vi "Periodic Tasks.vi"(8 "error in":errorcluster) -> ()   [LabVIEW 2018]
doc: "This VI runs in parallel to other tasks. It can contain as many user-defined periodic loops as you need. These can carry out PID or other sorts of timed response."
uses:
  <vilib>/Rock Robotics/WPI/ThirdParty/sensors/navX/_TypeDefs/Flags/Z900_navX_Flags_OpStatusTypeDef.ctl
  <vilib>/Rock Robotics/WPI/ThirdParty/sensors/navX/_TypeDefs/Flags/Z900_navX_Flags_CalibrationStatusTypeDef.ctl
  SwerveRotationCalibrate.ctl
  <vilib>/Rock Robotics/WPI/ThirdParty/Phoenix-LabVIEW/Motor Controller/Controls/CTRE_Phoenix_MotorControl_NeutralMode.ctl
  <vilib>/Rock Robotics/WPI/ThirdParty/Phoenix-LabVIEW/Motor Controller/Controls/CTRE_Phoenix_MotorControl_ControlMode.ctl
  <vilib>/Rock Robotics/WPI/ThirdParty/Phoenix-LabVIEW/Motor Controller/Controls/CTRE_Phoenix_MotorControl_FeedbackDevice.ctl
  HatchModes.ctl
  ElevBasePos.ctl
  ElevModes.ctl
  SequenceActions.ctl
  d8969dce-e83f-414b-ab1b-b6caec8a5545.vi
  83e91fab-fc29-4c7d-8b1e-156214dcbbb8.vi
  a102eae3-c5ed-494b-96cc-72fbbd712b4d.vi
  <vilib>/Rock Robotics/WPI/Utilities/WPI_GetSetVariantRefNum.vi
  <vilib>/Rock Robotics/Network Tables/NT Read Boolean.vi
  Robot Global Data.vi
  <vilib>/Rock Robotics/Network Tables/NT Write Number.vi
  <vilib>/Rock Robotics/Network Tables/NT Write String.vi
  <vilib>/Rock Robotics/Network Tables/NT Write Boolean.vi
panel:
  in  "Calibration Status":T1=3 items=["IMU_CAL_STATE_MASK"=3, "IMU_CAL_STATE_INPROGRESS"=0, "IMU_CAL_STATE_ACCUMULATE"=1, "IMU_CAL_STATE_COMPLETE"=2]
  in  "OP Status":T2 items=["INITIALIZING", "SELFTEST_IN_PROGRESS", "ERROR", "IMU_AUTOCAL_IN_PROGRESS", "NORMAL"]
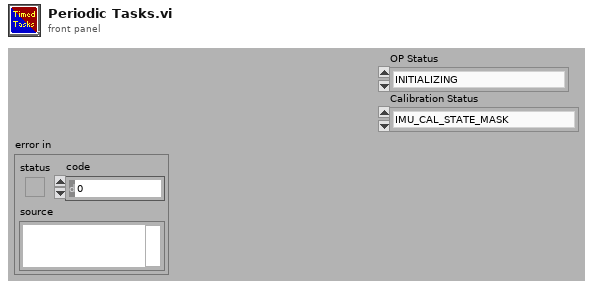
[diagram p1: front panel]
types:
  T1 = typedef "Z900_navX_Flags_CalibrationStatusTypeDef.ctl" = u8
  T2 = typedef "Z900_navX_Flags_OpStatusTypeDef.ctl" = u8
  T3 = typedef "HatchModes.ctl" = enum16{"Travel", "PickPlaceShip", "PlaceRocket"}
  T4 = typedef "SwerveRotationCalibrate.ctl" = enum16{"Calibrate", "Home", "ManualHome", "ResetQuad", "Drive"}
  T5 = typedef "CTRE_Phoenix_MotorControl_NeutralMode.ctl" = enum8{"EEPROMSetting", "Override to Coast", "Override to Brake"}
  T6 = typedef "CTRE_Phoenix_MotorControl_ControlMode.ctl" = u16
  T7 = typedef "CTRE_Phoenix_MotorControl_FeedbackDevice.ctl" = i8
  T8 = cluster{"T0":u32, "Mode":T4, "Rotation Neutral Mode":T5, "Rotation Control Mode":T6, "Feedback Device":T7}
  T9 = cluster{"Update Rate Hz":u8, "Accelerometer Full-Scale Range":u8, "Gyro Full-Scale Range":u16, "OP Status":T2, "Calibration Status":T1, "Sensor Status":cluster{"MOVING":bool, "YAW_STABLE":bool, "MAG_DISTURBANCE":bool, "ALTITUDE_VALID":bool, "SEALEVEL_PRESS_SET":bool, "FUSED_HEADING_VALID":bool}, "Self Test Status":cluster{"Gyro Passed":bool, "Accel Passed":bool, "Mag Passed":bool, "Baro Passed":bool, "Complete":bool}}
  T10 = typedef "ElevModes.ctl" = enum16{"Manual", "Auto"}
  T11 = typedef "ElevBasePos.ctl" = enum16{"NoChange", "ShipHatch", "RocketHatch", "Carry", "Cargo"}
  T12 = typedef "WPI_JoystickDevRef.ctl" = cluster{"Device":T13}
  T13 = typedef "WPI_JoystickDeviceEnum.ctl" = enum16{"USB 0", "USB 1", "USB 2", "USB 3", "USB 4", "USB 5"}
  T14 = typedef "SequenceActions.ctl" = enum16{"HatchLatch", "MoveElev", "Ready"}
  T15 = typedef "WPI_DriverStationRobotMode2.ctl" = enum16{"Autonomous Disabled", "Autonomous Enabled", "Teleop Disabled", "Teleop Enabled", "Disconnected", "Finish", "Test Disabled", "Test Enabled", "Emergency Stopped"}
  T16 = cluster{"Buttons[0]":bool, "Buttons[1]":bool, "Buttons[2]":bool, "Buttons[3]":bool, "Buttons[4]":bool, "Buttons[5]":bool, "Buttons[6]":bool, "Buttons[7]":bool, "Buttons[8]":bool, "Buttons[9]":bool, "Buttons[10]":bool, "Buttons[11]":bool, "Buttons[12]":bool}
  T17 = cluster{"Motor1":cluster{"P":dbl, "I":dbl, "D":dbl}, "Motor3":cluster{"P":dbl, "I":dbl, "D":dbl}, "Motor2":cluster{"P":dbl, "I":dbl, "D":dbl}, "Motor4":cluster{"P":dbl, "I":dbl, "D":dbl}}
  T18 = typedef "WPI_CompressorDevRef.ctl" = cluster{"DevStatus":errorcluster, "Pneumatics Control Module":u8}
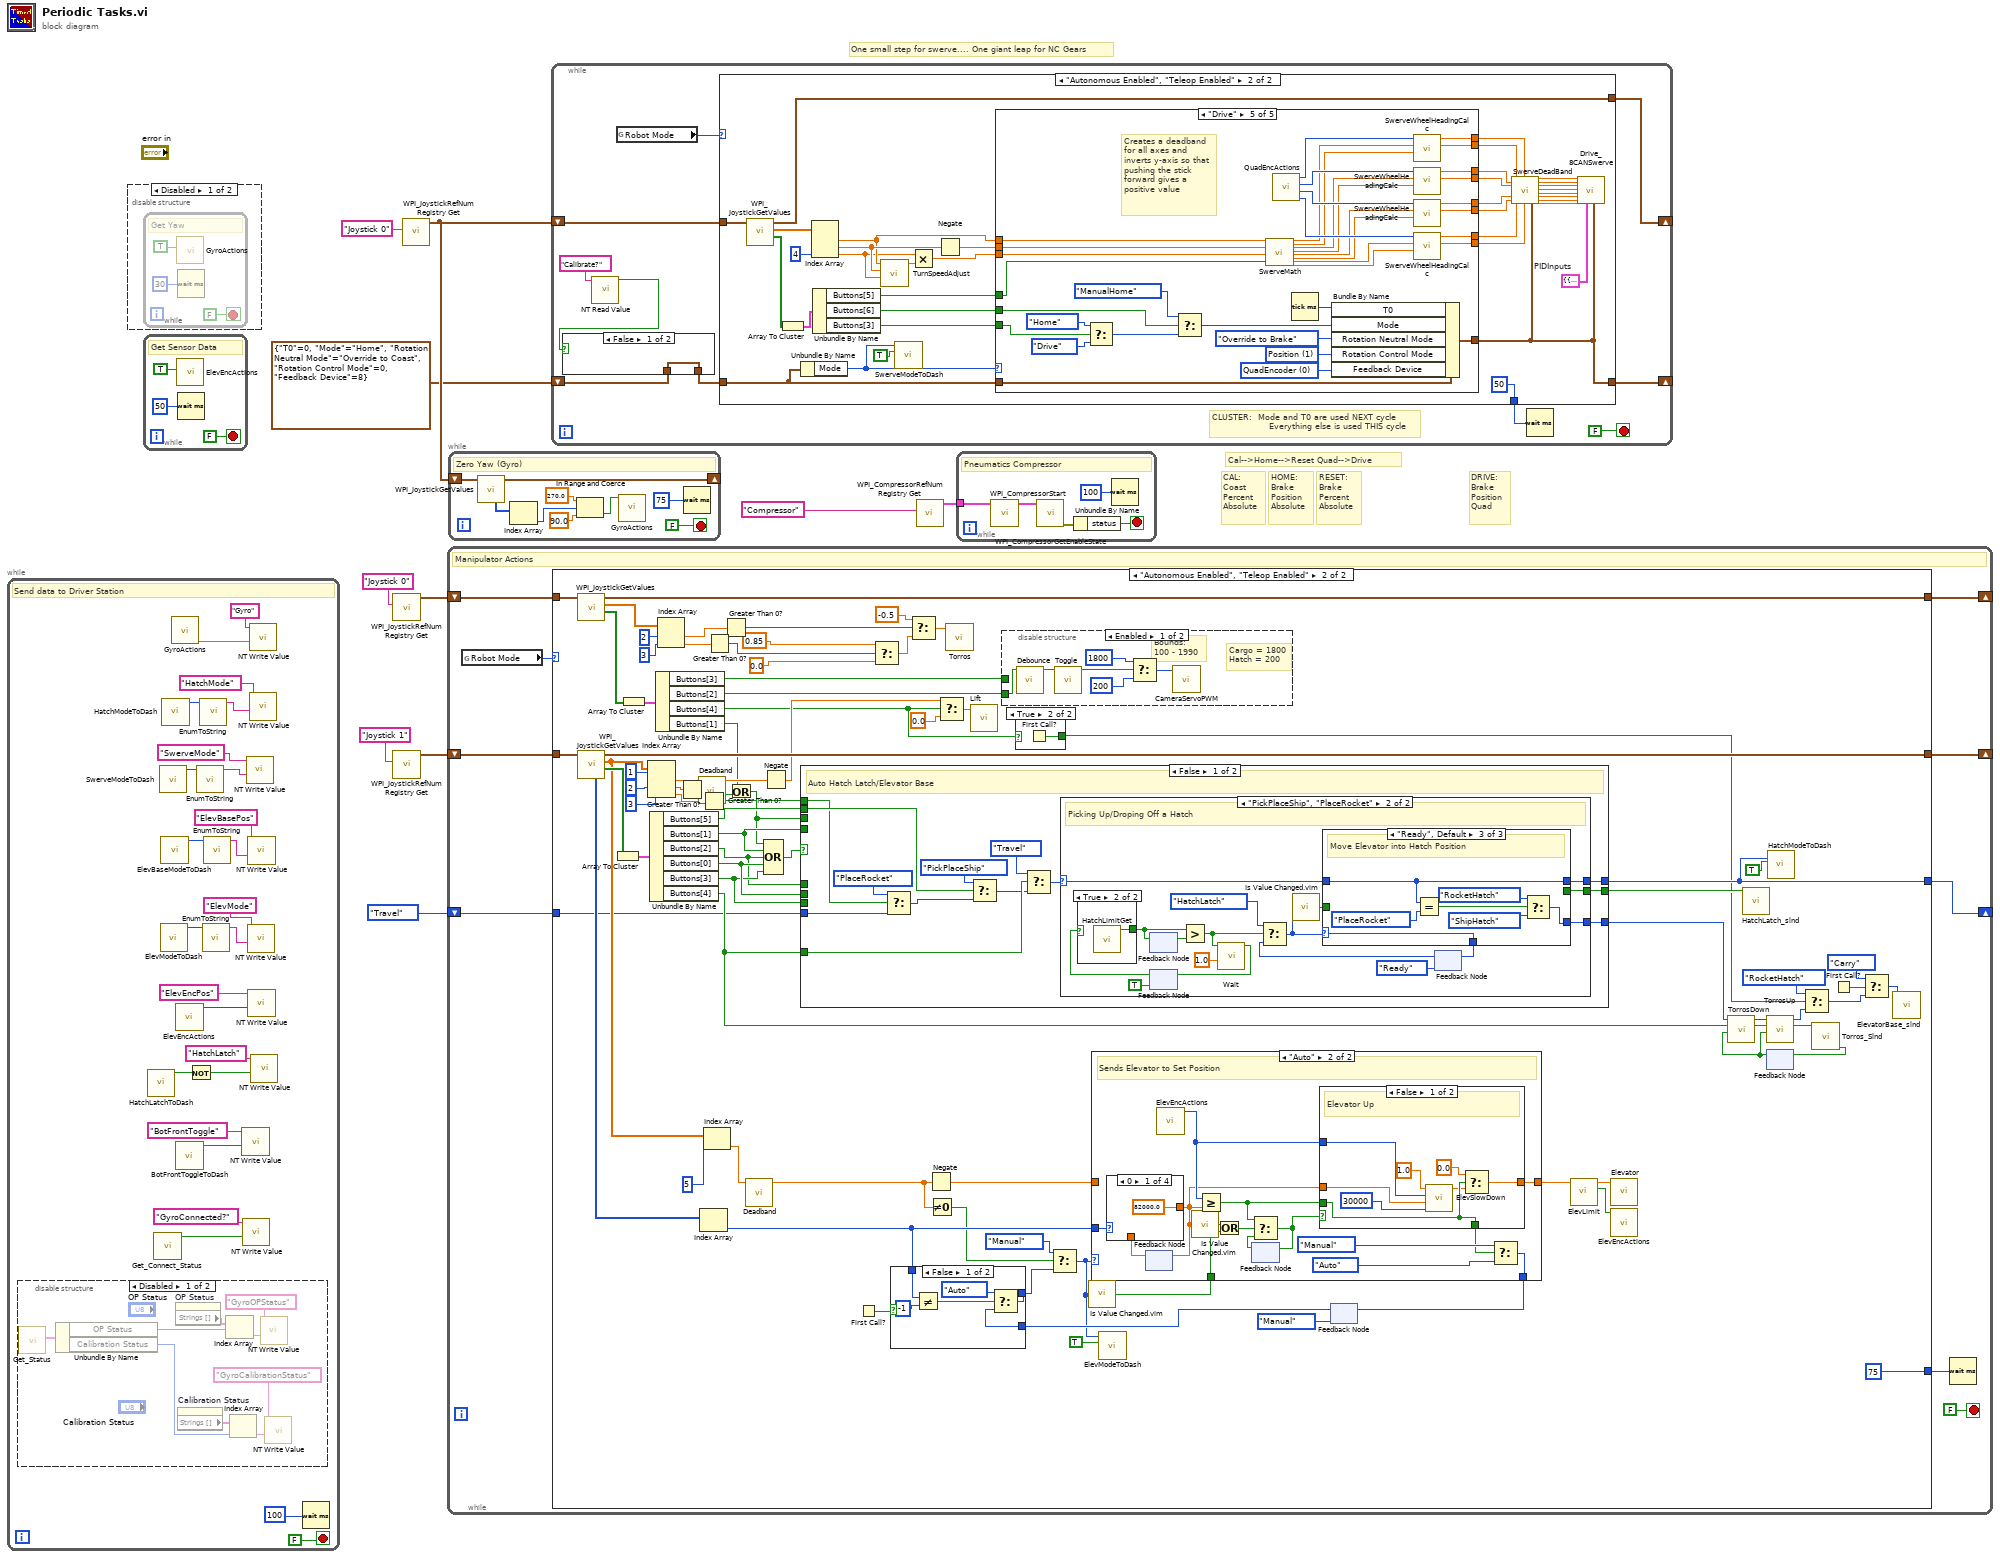
[diagram p0: block diagram]
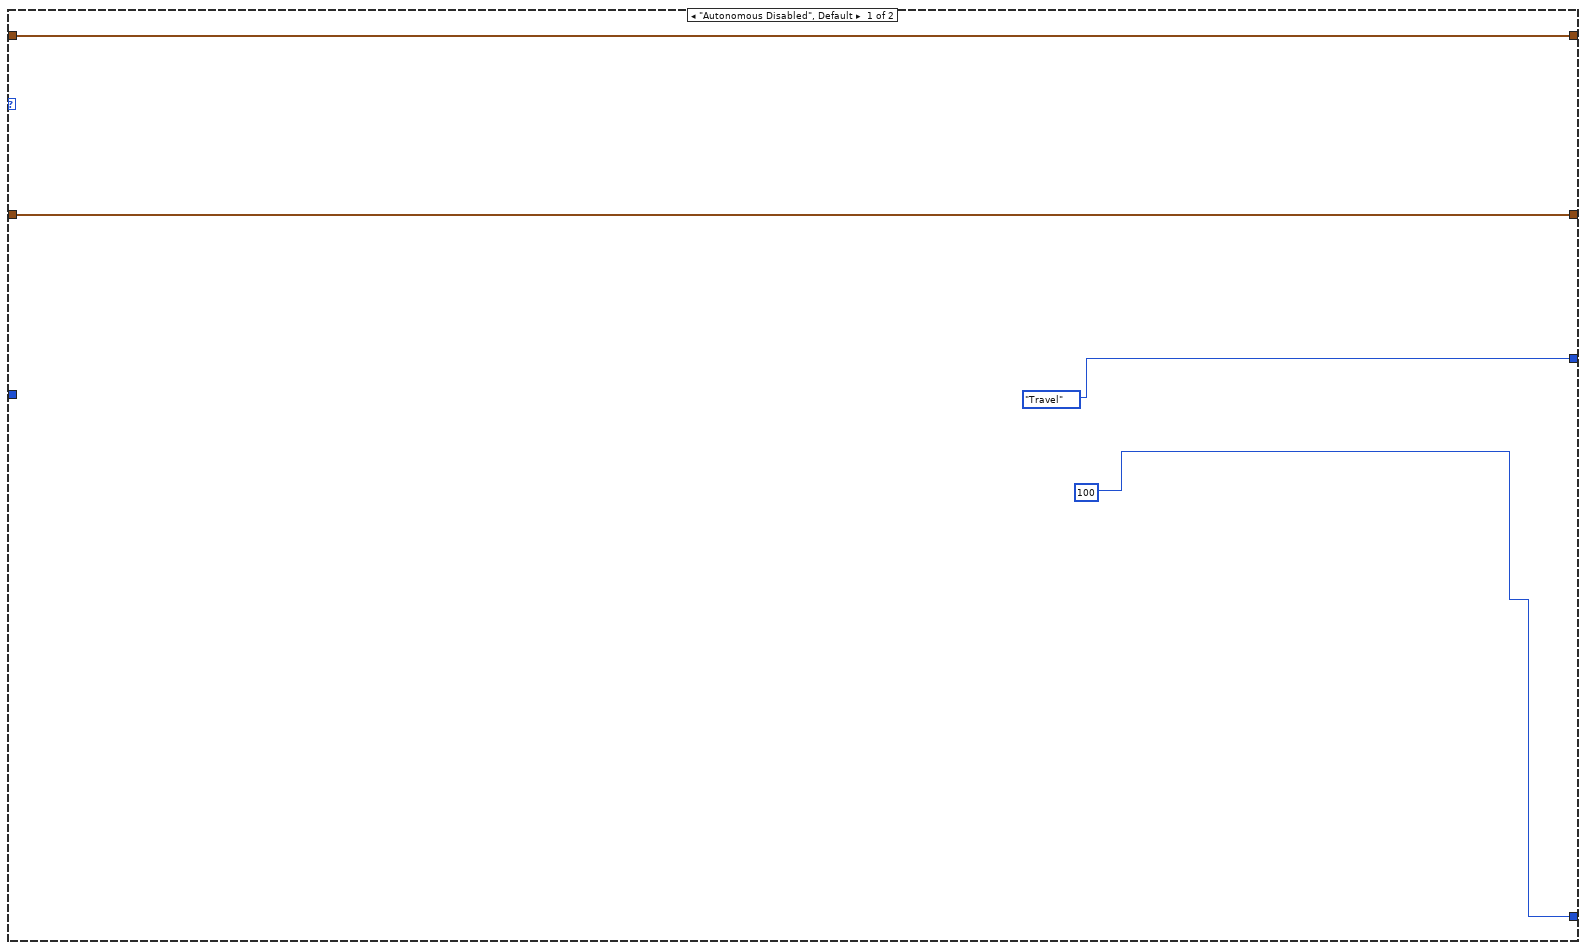
[diagram p3: hidden frame]
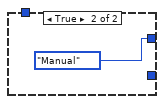
[diagram p4: hidden frame]
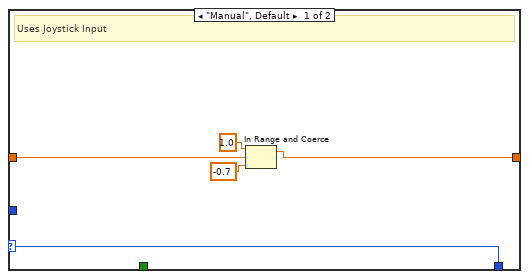
[diagram p5: hidden frame]
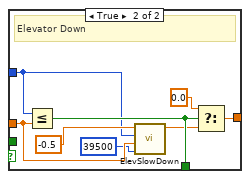
[diagram p6: hidden frame]
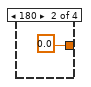
[diagram p7: hidden frame]
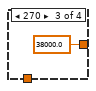
[diagram p8: hidden frame]
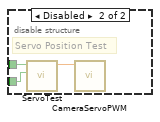
[diagram p11: hidden frame]
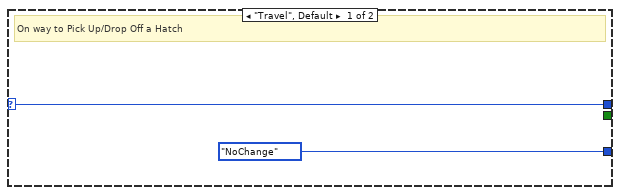
[diagram p12: hidden frame]
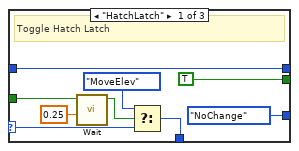
[diagram p14: hidden frame]
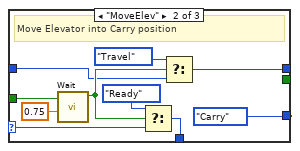
[diagram p15: hidden frame]
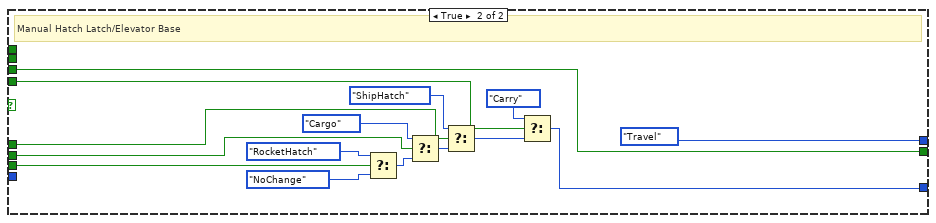
[diagram p16: hidden frame]
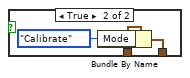
[diagram p17: hidden frame]
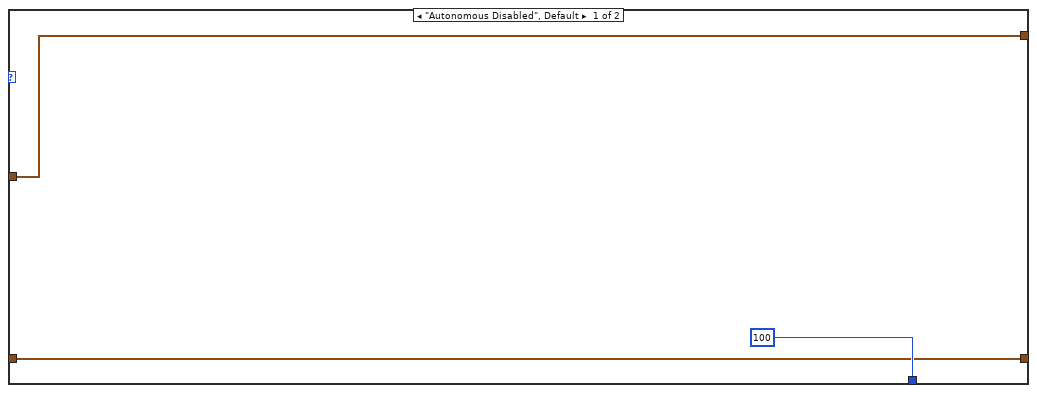
[diagram p18: hidden frame]
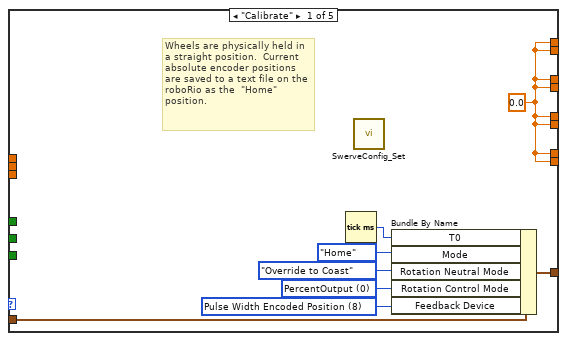
[diagram p19: hidden frame]
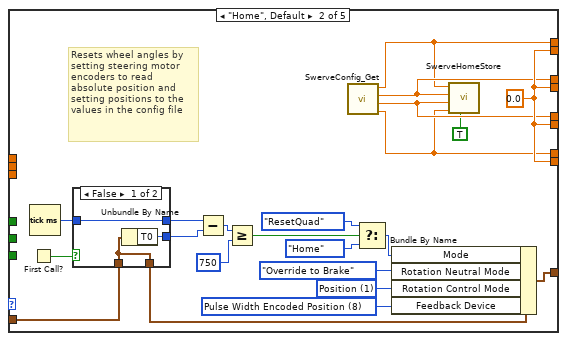
[diagram p20: hidden frame]
diagram:
  # "One small step for swerve.... One giant leap for NC Gears"
  # "DRIVE:\nBrake\nPosition\nQuad"
  # "RESET:\nBrake\nPercent\nAbsolute"
  # "HOME:\nBrake\nPosition\nAbsolute"
  # "Cal-->Home-->Reset Quad-->Drive"
  # "CAL:\nCoast\nPercent\nAbsolute"
  n1 = while {
    stop <- FALSE stop-if-true
    # "Send data to Driver Station"
    n2 = disable-structure shown="Disabled" {
      frame Disabled {
        n3 = call <vilib>:"Get_Status.vi"() -> ("Status"=w42:T9)  [unwired: 11 in]
        n4 = Unbundle By Name(w42) -> ("OP Status"=w40:T2, "Calibration Status"=w38:T1)
        n5 = property on="OP Status" class="Ring (strict)"() -> ("Strings []"=w41:string[])  [unwired: 2 in, 2 out]
        n6 = property on="Calibration Status" class="Ring (strict)"() -> ("Strings []"=w37:string[])  [unwired: 2 in, 2 out]
        n7 = Index Array(array=w41, index=w40) -> (element=w39:string)
        n8 = Index Array(array=w37, index=w38) -> (element=w36:string)
        n9 = call-poly <vilib>:"NT Write Value.vi"("String"=w39, "Name"="GyroOPStatus") -> ()  [unwired: 9 in, 1 out]
        n10 = call-poly <vilib>:"NT Write Value.vi"("String"=w36, "Name"="GyroCalibrationStatus") -> ()  [unwired: 9 in, 1 out]
      }
      frame Enabled {
      }
    }
    n11 = call "HatchLatchToDash.vi"() -> ("HatchLatchOut"=w11:bool)  [unwired: 11 in]
    n12 = call <vilib>:"Get_Connect_Status.vi"() -> ("Connected"=w19:bool)  [unwired: 11 in]
    n13 = call "SwerveModeToDash.vi"() -> ("SwerveModeOut"=w27:T4)  [unwired: 11 in]
    n14 = call "ElevModeToDash.vi"() -> ("ElevModeOut"=w17:T10)  [unwired: 11 in]
    n15 = call "ElevBaseModeToDash.vi"() -> ("ElevBasePosOut"=w22:T11)  [unwired: 11 in]
    n16 = call "HatchModeToDash.vi"() -> ("HatchModeOut"=w30:T3)  [unwired: 11 in]
    n17 = call "GyroActions.vi"() -> ("Yaw"=w18:dbl)  [unwired: 10 in, 1 out]
    n18 = call "ElevEncActions.vi"() -> ("ElevEncPos"=w24:i32)  [unwired: 11 in]
    n19 = call "BotFrontToggleToDash.vi"() -> ("FrontToggleOut"=w14:bool)  [unwired: 11 in]
    n20 = Not(x=w11) -> (.not. x?=w12:bool)
    n21 = call "EnumToString.vi"("Enum"=w27) -> ("String"=w26:string)  [unwired: 10 in]
    n22 = call "EnumToString.vi"("Enum"=w30) -> ("String"=w29:string)  [unwired: 10 in]
    n23 = call "EnumToString.vi"("Enum"=w17) -> ("String"=w16:string)  [unwired: 10 in]
    n24 = call "EnumToString.vi"("Enum"=w22) -> ("String"=w31:string)  [unwired: 10 in]
    n25 = call-poly <vilib>:"NT Write Value.vi"("Boolean"=w14, "Name"="BotFrontToggle") -> ()  [unwired: 9 in, 1 out]
    n26 = call-poly <vilib>:"NT Write Value.vi"("Boolean"=w19, "Name"="GyroConnected?") -> ()  [unwired: 9 in, 1 out]
    n27 = call-poly <vilib>:"NT Write Value.vi"("String"=w26, "Name"="SwerveMode") -> ()  [unwired: 9 in, 1 out]
    n28 = call-poly <vilib>:"NT Write Value.vi"("String"=w16, "Name"="ElevMode") -> ()  [unwired: 9 in, 1 out]
    n29 = call-poly <vilib>:"NT Write Value.vi"("String"=w31, "Name"="ElevBasePos") -> ()  [unwired: 9 in, 1 out]
    n30 = call-poly <vilib>:"NT Write Value.vi"("Numeric"=w24, "Name"="ElevEncPos") -> ()  [unwired: 9 in, 1 out]
    n31 = call-poly <vilib>:"NT Write Value.vi"("Numeric"=w18, "Name"="Gyro") -> ()  [unwired: 9 in, 1 out]
    n32 = call-poly <vilib>:"NT Write Value.vi"("String"=w29, "Name"="HatchMode") -> ()  [unwired: 9 in, 1 out]
    n33 = call-poly <vilib>:"NT Write Value.vi"("Boolean"=w12, "Name"="HatchLatch") -> ()  [unwired: 9 in, 1 out]
    n34 = Wait (ms)(milliseconds to wait=u32 100 ("millisecond timer value")) -> ()  [unwired: 1 out]
  }
  n35 = disable-structure shown="Disabled" {
    frame Disabled {
      n36 = while {
        stop <- FALSE stop-if-true
        # "Get Yaw"
        n37 = call "GyroActions.vi"("Update?"=TRUE ("Zero")) -> ()  [unwired: 9 in, 2 out]
        n38 = Wait (ms)(milliseconds to wait=u32 30) -> ()  [unwired: 1 out]
      }
    }
    frame Enabled {
    }
  }
  n39 = while {
    stop <- FALSE stop-if-true
    # "Get Sensor Data"
    n40 = call "ElevEncActions.vi"("Update?"=TRUE ("Zero")) -> ()  [unwired: 10 in, 1 out]
    n41 = Wait (ms)(milliseconds to wait=u32 50) -> ()  [unwired: 1 out]
  }
  n42 = call <vilib>:"WPI_JoystickRefNum Registry Get.vi"("refnum name"="Joystick 0") -> ("JoystickDevRef"=w2:T12)  [unwired: 1 in, 9 out]
  n43 = call <vilib>:"WPI_JoystickRefNum Registry Get.vi"("refnum name"="Joystick 1") -> ("JoystickDevRef"=w6:T12)  [unwired: 1 in, 9 out]
  n44 = call <vilib>:"WPI_JoystickRefNum Registry Get.vi"("refnum name"="Joystick 0") -> ("JoystickDevRef"=w9:T12)  [unwired: 1 in, 9 out]
  n45 = while {
    shift-right: [w53] -> _
    shift-left: HatchModes."Travel" -> [w54]
    shift-right: [w52] -> _
    shift-left: w6 -> [w58]
    shift-right: [w51] -> _
    shift-left: w2 -> [w55]
    stop <- FALSE stop-if-true
    # "Manipulator Actions"
    n46 = global read "Robot Global Data.vi" "Robot Mode"() -> (w59:T15)
    n47 = case shown="\"Autonomous Enabled\", \"Teleop Enabled\"" w59 {
      tunnel: w58 -> [w61 w144]
      tunnel: [u32 100 ("milliseconds to wait") u32 75 ("milliseconds to wait")] -> w56
      tunnel: w55 -> [w60 w138]
      tunnel: w54 -> [_ w93]
      tunnel: [HatchModes."Travel" w106] -> w53
      tunnel: [w61 w101] -> w52
      tunnel: [w60 w64] -> w51
      frame "Autonomous Disabled", Default {
      }
      frame "Autonomous Enabled", "Teleop Enabled" {
        n48 = call <vilib>:"WPI_JoystickGetValues.vi"("JoystickDevRef"=w138) -> ("Buttons"=w139:bool[], "Axes"=w128:dbl[], "JoystickDevRef"=w64:T12)  [unwired: 6 in, 2 out]
        n49 = call <vilib>:"WPI_JoystickGetValues.vi"("JoystickDevRef"=w144) -> ("Buttons"=w143:bool[], "Axes"=w102:dbl[], "JoystickDevRef"=w101:T12, "POVs"=w141:i16[])  [unwired: 6 in, 1 out]
        n50 = Array To Cluster(array=w143) -> (cluster=w145:T16)
        n51 = Array To Cluster(array=w139) -> (cluster=w140:T16)
        n52 = Index Array(array=w102, index #1=1 ("index"), index #2=2 ("index"), index #3=3 ("index")) -> (element #1=w100:dbl, element #2=w89:dbl, element #3=w70:dbl)
        n53 = Unbundle By Name(w145) -> ("Buttons[5]"=w114:bool, "Buttons[1]"=w136:bool, "Buttons[2]"=w104:bool, "Buttons[0]"=w135:bool, "Buttons[3]"=w134:bool, "Buttons[4]"=w94:bool)
        n54 = Unbundle By Name(w140) -> ("Buttons[3]"=w91:bool, "Buttons[2]"=w92:bool, "Buttons[4]"=w84:bool, "Buttons[1]"=w65:bool)
        n55 = Index Array(array=w128, index #1=2 ("index"), index #2=3 ("index")) -> (element #1=w124:dbl, element #2=w125:dbl)
        n56 = Greater Than 0?(x=w89) -> (x > 0?=w88:bool)
        n57 = call "Deadband.vi"("Input"=w100) -> ("Output"=w71:dbl)  [unwired: 6 in]
        n58 = Index Array(array=w141) -> (element=w130:i16)  [unwired: 1 in]
        n59 = Greater Than 0?(x=w70) -> (x > 0?=w69:bool)
        n60 = Index Array(array=w102, index=5) -> (element=w115:dbl)
        n61 = Greater Than 0?(x=w125) -> (x > 0?=w122:bool)
        n62 = Greater Than 0?(x=w124) -> (x > 0?=w123:bool)
        n63 = Or(x=w65, y=w88) -> (x .or. y?=w87:bool)
        n64 = call "Deadband.vi"("Input"=w115) -> ("Output"=w132:dbl)  [unwired: 6 in]
        n65 = Negate(x=w71) -> (-x=w98:dbl)
        n66 = Compound Arithmetic op=OR(w87, w136, w104, w135, w134) -> (w137:bool)
        n67 = case shown="False" w137 {
          tunnel: w93 -> [w205 _]
          tunnel: [w215 HatchModes."Travel"] -> w106
          tunnel: [w214 w275] -> w133
          tunnel: w87 -> [_ w275]
          tunnel: w136 -> [_ w274]
          tunnel: w104 -> [_ w273]
          tunnel: w135 -> [_ w272]
          tunnel: w134 -> [_ w271]
          tunnel: w114 -> [w212 _]
          tunnel: [w211 w262] -> w111
          tunnel: w94 -> [w210 _]
          tunnel: w69 -> [w203 _]
          frame False {
            # "Auto Hatch Latch/Elevator Base"
            n68 = Select(t=HatchModes."PlaceRocket", s=w203, f=w205) -> (s? t:f=w204:T3)
            n69 = Select(t=HatchModes."PickPlaceShip", s=w212, f=w204) -> (s? t:f=w208:T3)
            n70 = Select(t=HatchModes."Travel", s=w210, f=w208) -> (s? t:f=w207:T3)
            n71 = case shown="\"PickPlaceShip\", \"PlaceRocket\"" w207 {
              selector: w207 -> [w217 w234]
              tunnel: [w217 w233] -> w215
              tunnel: [_ w232] -> w214
              tunnel: [ElevBasePos."NoChange" w225] -> w211
              frame "Travel", Default {
                # "On way to Pick Up/Drop Off a Hatch"
              }
              frame "PickPlaceShip", "PlaceRocket" {
                # "Picking Up/Droping Off a Hatch"
                n72 = feedback #1() -> (w220:bool)  [unwired: 1 in]
                n73 = feedback #2(TRUE ("Completed")) -> (w222:bool)
                n74 = case shown="True" w222 {
                  tunnel: [_ w235] -> w218
                  frame False {
                  }
                  frame True {
                    n75 = call "HatchLimitGet.vi"() -> ("Pressed?"=w235:bool)  [unwired: 11 in]
                  }
                }
                n76 = feedback-in #1(w218) -> ()
                n77 = Greater?(x=w218, y=w220) -> (0:w219:bool)
                n78 = call "Wait.vi"("Target Time (s)"=1.0, "Start Timer?"=w219) -> ("Completed"=w223:bool)  [unwired: 8 in, 1 out]
                n79 = feedback-in #2(w223) -> ()
                n80 = feedback #3(SequenceActions."Ready" ("SequenceAction")) -> (w229:T14)
                n81 = Select(t=SequenceActions."HatchLatch" ("SequenceAction"), s=w219, f=w229) -> (s? t:f=w231:T14)
                n82 = call "Is Value Changed.vim"("value"=w231) -> ("changed or first call?"=w226:bool)
                n83 = case shown="\"Ready\", Default" w231 {
                  selector: w231 -> [w243 w254 w261]
                  tunnel: [w242 w253 w261] -> w230
                  tunnel: w234 -> [w241 w250 w255]
                  tunnel: [w241 w249 w255] -> w233
                  tunnel: [TRUE _ _] -> w232
                  tunnel: w226 -> [w238 w247 _]
                  tunnel: [ElevBasePos."NoChange" ElevBasePos."Carry" w258] -> w225
                  frame "HatchLatch" {
                    # "Toggle Hatch Latch"
                    n84 = call "Wait.vi"("Target Time (s)"=0.25, "Start Timer?"=w238) -> ("Completed"=w244:bool)  [unwired: 8 in, 1 out]
                    n85 = Select(t=SequenceActions."MoveElev" ("SequenceAction"), s=w244, f=w243) -> (s? t:f=w242:T14)
                  }
                  frame "MoveElev" {
                    # "Move Elevator into Carry position"
                    n86 = call "Wait.vi"("Target Time (s)"=0.75, "Start Timer?"=w247) -> ("Completed"=w252:bool)  [unwired: 8 in, 1 out]
                    n87 = Select(t=SequenceActions."Ready" ("SequenceAction"), s=w252, f=w254) -> (s? t:f=w253:T14)
                    n88 = Select(t=HatchModes."Travel", s=w252, f=w250) -> (s? t:f=w249:T3)
                  }
                  frame "Ready", Default {
                    # "Move Elevator into Hatch Position"
                    n89 = Equal?(x=w255, y=HatchModes."PlaceRocket") -> (x = y?=w257:bool)
                    n90 = Select(t=ElevBasePos."RocketHatch", s=w257, f=ElevBasePos."ShipHatch") -> (s? t:f=w258:T11)
                  }
                }
                n91 = feedback-in #3(w230) -> ()
              }
            }
          }
          frame True {
            # "Manual Hatch Latch/Elevator Base"
            n92 = Select(t=ElevBasePos."RocketHatch", s=w271, f=ElevBasePos."NoChange") -> (s? t:f=w270:T11)
            n93 = Select(t=ElevBasePos."Cargo", s=w272, f=w270) -> (s? t:f=w269:T11)
            n94 = Select(t=ElevBasePos."ShipHatch", s=w273, f=w269) -> (s? t:f=w268:T11)
            n95 = Select(t=ElevBasePos."Carry", s=w274, f=w268) -> (s? t:f=w262:T11)
          }
        }
        n96 = First Call?() -> (First Call?: T/F=w66:bool)
        n97 = Select(t=0.85, s=w122, f=0.0) -> (s? t:f=w121:dbl)
        n98 = Select(t=-0.5, s=w123, f=w121) -> (s? t:f=w120:dbl)
        n99 = Negate(x=w132) -> (-x=w75:dbl)
        n100 = Not Equal To 0?(x=w132) -> (x != 0?=w76:bool)
        n101 = Select(t=w98, s=w84, f=0.0 ("t")) -> (s? t:f=w86:dbl)
        n102 = call "Torros.vi"("Power"=w120) -> ()  [unwired: 11 in]
        n103 = call "Lift.vi"("Power"=w86) -> ()  [unwired: 11 in]
        n104 = disable-structure shown="Enabled" {
          disable-tunnel: w92 -> [w195 w202]
          disable-tunnel: w91 -> [_ w201]
          frame Enabled {
            # "Cargo = 1800\nHatch = 200"
            # "Bounds: 100 - 1990"
            n105 = call "Debounce.vi"("booleanIn"=w195) -> ("booleanOut"=w196:bool)  [unwired: 10 in]
            n106 = call "Toggle.vi"("booleanIn"=w196) -> ("booleanOut"=w197:bool)  [unwired: 10 in]
            n107 = Select(t=1800, s=w197, f=200) -> (s? t:f=w194:i32)
            n108 = call "CameraServoPWM.vi"("Position"=w194) -> ()  [unwired: 11 in]
          }
          frame Disabled {
            # "Servo Position Test"
            n109 = call "ServoTest.vi"("Down"=w202, "Up"=w201) -> ("Angle"=w200:dbl)  [unwired: 9 in]
            n110 = call "CameraServoPWM.vi"("Position"=w200) -> ()  [unwired: 11 in]
          }
        }
        n111 = case shown="True" w84 {
          tunnel: [_ w193] -> w83
          frame False {
          }
          frame True {
            n112 = First Call?() -> (First Call?: T/F=w193:bool)
          }
        }
        n113 = feedback #4(ElevModes."Manual") -> (w77:T10)
        n114 = case shown="False" w66 {
          tunnel: w130 -> [w151 _]
          tunnel: [w150 ElevModes."Manual"] -> w79
          tunnel: w77 -> [w148 _]
          frame False {
            n115 = Not Equal?(x=w151, y=i16 -1) -> (x != y?=w146:bool)
            n116 = Select(t=ElevModes."Auto", s=w146, f=w148) -> (s? t:f=w150:T10)
          }
          frame True {
          }
        }
        n117 = Select(t=ElevModes."Manual", s=w76, f=w79) -> (s? t:f=w68:T10)
        n118 = call "Is Value Changed.vim"("value"=w68) -> ("changed or first call?"=w74:bool)
        n119 = case shown="\"Auto\"" w68 {
          selector: w68 -> [w157 _]
          tunnel: w130 -> [_ w172]
          tunnel: [w155 w171] -> w131
          tunnel: w75 -> [w156 _]
          tunnel: w74 -> [_ w163]
          tunnel: [w157 w158] -> w73
          frame "Manual", Default {
            # "Uses Joystick Input"
            n120 = In Range and Coerce(upper limit=1.0, x=w156, lower limit=-0.7) -> (coerced(x)=w155:dbl)  [unwired: 1 out]
          }
          frame "Auto" {
            # "Sends Elevator to Set Position"
            n121 = feedback #5() -> (w166:dbl)  [unwired: 1 in]
            n122 = case shown="0" w172 {
              tunnel: [82000.0 ("Target") 0.0 ("Target") 38000.0 ("Target") w192] -> w165
              tunnel: w166 -> [_ _ _ w192]
              frame 0 {
              }
              frame 180 {
              }
              frame 270 {
              }
              frame -1, Default {
              }
            }
            n123 = feedback-in #5(w165) -> ()
            n124 = call "ElevEncActions.vi"() -> ("ElevEncPos"=w167:i32)  [unwired: 11 in]
            n125 = call "Is Value Changed.vim"("value"=w165) -> ("changed or first call?"=w164:bool)
            n126 = Greater Or Equal?(x=w167, y=w165) -> (x >= y?=w168:bool)
            n127 = Or(x=w164, y=w163) -> (x .or. y?=w162:bool)
            n128 = feedback #6() -> (w170:bool)  [unwired: 1 in]
            n129 = Select(t=w168, s=w162, f=w170) -> (s? t:f=w169:bool)
            n130 = feedback-in #6(w169) -> ()
            n131 = case shown="False" w169 {
              tunnel: [w179 w187] -> w171
              tunnel: w165 -> [w175 w183]
              tunnel: w167 -> [w176 w184]
              tunnel: w168 -> [w178 _]
              tunnel: [w178 w186] -> w159
              frame False {
                # "Elevator Up"
                n132 = call "ElevSlowDown.vi"("SlowRange"=30000 ("y"), "Target"=w175, "Current"=w176, "ElevIn"=1.0) -> ("ElevOut"=w174:dbl)  [unwired: 7 in]
                n133 = Select(t=0.0, s=w178, f=w174) -> (s? t:f=w179:dbl)
              }
              frame True {
                # "Elevator Down"
                n134 = Less Or Equal?(x=w184, y=w183) -> (x <= y?=w186:bool)
                n135 = call "ElevSlowDown.vi"("SlowRange"=39500 ("y"), "Target"=w183, "Current"=w184, "ElevIn"=-0.5) -> ("ElevOut"=w182:dbl)  [unwired: 7 in]
                n136 = Select(t=0.0, s=w186, f=w182) -> (s? t:f=w187:dbl)
              }
            }
            n137 = Select(t=ElevModes."Manual", s=w159, f=ElevModes."Auto") -> (s? t:f=w158:T10)
          }
        }
        n138 = call "ElevModeToDash.vi"("Update?"=TRUE, "ElevModeIn"=w68) -> ()  [unwired: 9 in, 1 out]
        n139 = feedback-in #4(w73) -> ()
        n140 = call "ElevLimit.vi"("PowerIn"=w131) -> ("BotLimit"=w105:bool, "PowerOut"=w129:dbl)  [unwired: 8 in, 1 out]
        n141 = call "Elevator.vi"("Power"=w129) -> ()  [unwired: 11 in]
        n142 = call "ElevEncActions.vi"("Zero?"=w105) -> ()  [unwired: 10 in, 1 out]
        n143 = call "HatchLatch_slnd.vi"("Toggle?"=w133) -> ()  [unwired: 11 in]
        n144 = feedback #7() -> (w109:bool)  [unwired: 1 in]
        n145 = call "TorrosDown.vi"("TorrosCurrPos"=w109, "TorrosButton"=w94, "ElevBasePosIn"=w111) -> ("TorrosOut"=w112:bool, "ElevBasePosOut"=w110:T11)  [unwired: 7 in]
        n146 = call "TorrosUp.vi"("TorrosCurrPos"=w109, "TorrosIn"=w112, "ElevBasePosIn"=w110) -> ("TorrosOut"=w113:bool, "ElevBasePosOut"=w82:T11)  [unwired: 7 in]
        n147 = call "HatchModeToDash.vi"("Update?"=TRUE, "HatchModeIn"=w106) -> ()  [unwired: 9 in, 1 out]
        n148 = Select(t=ElevBasePos."RocketHatch", s=w83, f=w82) -> (s? t:f=w81:T11)
        n149 = call "Torros_Slnd.vi"("Toggle?"=w113) -> ("CurrState"=w108:bool)  [unwired: 10 in]
        n150 = feedback-in #7(w108) -> ()
        n151 = First Call?() -> (First Call?: T/F=w96:bool)
        n152 = Select(t=ElevBasePos."Carry", s=w96, f=w81) -> (s? t:f=w97:T11)
        n153 = call "ElevatorBase_slnd.vi"("ElevBasePosIn"=w97) -> ()  [unwired: 11 in]
      }
    }
    n154 = Wait (ms)(milliseconds to wait=w56) -> ()  [unwired: 1 out]
  }
  n155 = while {
    shift-right: [w278] -> _
    shift-left: w9 -> [w285]
    stop <- FALSE stop-if-true
    # "Zero Yaw (Gyro)"
    n156 = call <vilib>:"WPI_JoystickGetValues.vi"("JoystickDevRef"=w285) -> ("JoystickDevRef"=w278:T12, "POVs"=w283:i16[])  [unwired: 6 in, 3 out]
    n157 = Index Array(array=w283) -> (element=w282:i16)  [unwired: 1 in]
    n158 = In Range and Coerce(upper limit=270.0, x=w282, lower limit=90.0) -> (In Range?=w281:bool)  [unwired: 1 out]
    n159 = call "GyroActions.vi"("Zero"=w281) -> ()  [unwired: 9 in, 2 out]
    n160 = Wait (ms)(milliseconds to wait=u32 75) -> ()  [unwired: 1 out]
  }
  n161 = while {
    shift-right: [w293] -> _
    shift-left: w9 -> [w294]
    shift-right: [w292] -> _
    shift-left: T8 {"T0"=0, "Mode"=enum."Home", "Rotation Neutral Mode"=enum."Override to Coast", "Rotation Control Mode"=0, "Feedback Device"=8} ("RotationSettings") -> [w288]
    stop <- FALSE stop-if-true
    # "CLUSTER:  Mode and T0 are used NEXT cycle\n                   Everything else is used THIS cycle"
    n162 = call-poly <vilib>:"NT Read Value.vi"("Name"="Calibrate?") -> ("Boolean"=w286:bool)  [unwired: 9 in, 1 out]
    n163 = case shown="False" w286 {
      tunnel: w288 -> [w296 w299]
      tunnel: [w296 w298] -> w287
      frame False {
      }
      frame True {
        n164 = Bundle By Name(cluster=w299, "Mode"=SwerveRotationCalibrate."Calibrate") -> (w298:T8)
      }
    }
    n165 = global read "Robot Global Data.vi" "Robot Mode"() -> (w290:T15)
    n166 = case shown="\"Autonomous Enabled\", \"Teleop Enabled\"" w290 {
      tunnel: w294 -> [w300 w339]
      tunnel: [w300 w338] -> w293
      tunnel: [w301 w314] -> w292
      tunnel: w287 -> [w301 w333]
      tunnel: [u32 100 ("milliseconds to wait") u32 50 ("milliseconds to wait")] -> w291
      frame "Autonomous Disabled", Default {
      }
      frame "Autonomous Enabled", "Teleop Enabled" {
        w334 = T17 {"Motor1"={"P"=4.0, "I"=0.0, "D"=64.0}, "Motor3"={"P"=4.0, "I"=0.0, "D"=64.0}, "Motor2"={"P"=4.0, "I"=0.0, "D"=64.0}, "Motor4"={"P"=4.0, "I"=0.0, "D"=64.0}}  # PIDInputs
        n167 = call <vilib>:"WPI_JoystickGetValues.vi"("JoystickDevRef"=w339) -> ("Buttons"=w336:bool[], "Axes"=w337:dbl[], "JoystickDevRef"=w338:T12)  [unwired: 6 in, 2 out]
        n168 = Array To Cluster(array=w336) -> (cluster=w335:T16)
        n169 = Unbundle By Name(w333) -> ("Mode"=w311:T4)
        n170 = Index Array(array=w337, index #3=4 ("index")) -> (element #1=w305:dbl, element #2=w306:dbl, element #3=w304:dbl)  [unwired: 2 in]
        n171 = Unbundle By Name(w335) -> ("Buttons[5]"=w303:bool, "Buttons[6]"=w308:bool, "Buttons[3]"=w312:bool)
        n172 = call "TurnSpeedAdjust.vi"("Turn"=w304, "Y"=w306, "X"=w305) -> ("TurnAdjusted"=w307:dbl)  [unwired: 8 in]
        n173 = call "SwerveModeToDash.vi"("Update?"=TRUE, "SwerveModeIn"=w311) -> ()  [unwired: 9 in, 1 out]
        n174 = Multiply(x=w304, y=w307) -> (x*y=w313:dbl)
        n175 = Negate(x=w306) -> (-x=w331:dbl)
        n176 = case shown="\"Drive\"" w311 {
          tunnel: [w341 w369 w394 w406 w443] -> w327
          tunnel: [w341 w349 w376 w401 w437] -> w330
          tunnel: [w341 w369 w394 w406 w441] -> w329
          tunnel: [w341 w352 w376 w402 w442] -> w328
          tunnel: [w341 w369 w394 w406 w447] -> w323
          tunnel: [w341 w350 w376 w404 w446] -> w324
          tunnel: [w341 w369 w394 w406 w445] -> w326
          tunnel: [w341 w351 w376 w403 w444] -> w325
          tunnel: w333 -> [w347 w354 w379 w410 w434]
          tunnel: [w345 w365 w390 w409 w432] -> w314
          tunnel: w312 -> [_ _ _ _ w429]
          tunnel: w331 -> [_ _ _ _ w425]
          tunnel: w313 -> [_ _ _ _ w424]
          tunnel: w305 -> [_ _ _ _ w423]
          tunnel: w308 -> [_ _ _ _ w413]
          tunnel: w303 -> [_ _ _ _ w411]
          frame "Calibrate" {
            w341 = 0.0 ("P")
            w344 = T6 0 items=["PercentOutput"=0, "Position"=1, "Velocity"=2, "Current"=3, "Follower"=5, "MotionProfile"=6, "MotionMagic"=7, "MotionProfileArc"=10, "Disabled"=15] ("Rotation Control Mode")
            w346 = T7 8 items=["None"=-1, "QuadEncoder"=0, "Analog"=2, "Tachometer"=4, "Pulse Width Encoded Position"=8, "Sensor Sum (S0 + S1)"=9, "Sensor Difference (D0 - D1)"=10, "Remote Source 0"=11, "Remote Source 1"=12, "Software Emulated"=15] ("Feedback Device")
            # "Wheels are physically held in a straight position.  Current absolute encoder positions are saved to a text file on the roboRio as the  \"Home\" position."
            n177 = Tick Count (ms)() -> (millisecond timer value=w340:u32)
            n178 = call "SwerveConfig_Set.vi"() -> ()  [unwired: 12 in]
            n179 = Bundle By Name(cluster=w347, "T0"=w340, "Mode"=SwerveRotationCalibrate."Home", "Rotation Neutral Mode"=CTRE_Phoenix_MotorControl_NeutralMode."Override to Coast", "Rotation Control Mode"=w344, "Feedback Device"=w346) -> (w345:T8)
          }
          frame "Home", Default {
            w367 = T6 1 items=["PercentOutput"=0, "Position"=1, "Velocity"=2, "Current"=3, "Follower"=5, "MotionProfile"=6, "MotionMagic"=7, "MotionProfileArc"=10, "Disabled"=15] ("Rotation Control Mode")
            w368 = T7 8 items=["None"=-1, "QuadEncoder"=0, "Analog"=2, "Tachometer"=4, "Pulse Width Encoded Position"=8, "Sensor Sum (S0 + S1)"=9, "Sensor Difference (D0 - D1)"=10, "Remote Source 0"=11, "Remote Source 1"=12, "Software Emulated"=15] ("Feedback Device")
            w369 = 0.0 ("P")
            # "Resets wheel angles by setting steering motor encoders to read absolute position and setting positions to the values in the config file"
            n180 = First Call?() -> (First Call?: T/F=w358:bool)
            n181 = Tick Count (ms)() -> (millisecond timer value=w357:u32)
            n182 = case shown="False" w358 {
              tunnel: w354 -> [w371 w375]
              tunnel: w357 -> [w372 w373]
              tunnel: [w372 w373] -> w356
              tunnel: [w371 w374] -> w355
              tunnel: [w370 w373] -> w353
              frame False {
                n183 = Unbundle By Name(w371) -> ("T0"=w370:u32)
              }
              frame True {
                n184 = Bundle By Name(cluster=w375, "T0"=w373) -> (w374:T8)
              }
            }
            n185 = Subtract(x=w356, y=w353) -> (x-y=w361:u32)
            n186 = Greater Or Equal?(x=w361, y=u32 750) -> (x >= y?=w360:bool)
            n187 = call "SwerveConfig_Get.vi"() -> ("RearRightHome"=w350:dbl, "RearLeftHome"=w351:dbl, "FrontRightHome"=w352:dbl, "FrontLeftHome"=w349:dbl)  [unwired: 8 in]
            n188 = Select(t=SwerveRotationCalibrate."ResetQuad" ("Mode"), s=w360, f=SwerveRotationCalibrate."Home" ("Mode")) -> (s? t:f=w364:T4)
            n189 = Bundle By Name(cluster=w355, "Mode"=w364, "Rotation Neutral Mode"=CTRE_Phoenix_MotorControl_NeutralMode."Override to Brake", "Rotation Control Mode"=w367, "Feedback Device"=w368) -> (w365:T8)
            n190 = call "SwerveHomeStore.vi"("Update?"=TRUE, "RearRightHomeIn"=w350, "RearLeftHomeIn"=w351, "FrontRightHomeIn"=w352, "FrontLeftHomeIn"=w349) -> ()  [unwired: 3 in, 4 out]
          }
          frame "ManualHome" {
            w376 = 0.0 ("P")
            w392 = T6 1 items=["PercentOutput"=0, "Position"=1, "Velocity"=2, "Current"=3, "Follower"=5, "MotionProfile"=6, "MotionMagic"=7, "MotionProfileArc"=10, "Disabled"=15] ("Rotation Control Mode")
            w393 = T7 8 items=["None"=-1, "QuadEncoder"=0, "Analog"=2, "Tachometer"=4, "Pulse Width Encoded Position"=8, "Sensor Sum (S0 + S1)"=9, "Sensor Difference (D0 - D1)"=10, "Remote Source 0"=11, "Remote Source 1"=12, "Software Emulated"=15] ("Feedback Device")
            w394 = 0.0 ("P")
            # "Resets wheel angles by setting steering motor encoders to read absolute position and setting positions to the values in the config file"
            n191 = First Call?() -> (First Call?: T/F=w383:bool)
            n192 = Tick Count (ms)() -> (millisecond timer value=w382:u32)
            n193 = case shown="False" w383 {
              tunnel: w379 -> [w396 w400]
              tunnel: w382 -> [w397 w398]
              tunnel: [w397 w398] -> w381
              tunnel: [w396 w399] -> w380
              tunnel: [w395 w398] -> w378
              frame False {
                n194 = Unbundle By Name(w396) -> ("T0"=w395:u32)
              }
              frame True {
                n195 = Bundle By Name(cluster=w400, "T0"=w398) -> (w399:T8)
              }
            }
            n196 = Subtract(x=w381, y=w378) -> (x-y=w386:u32)
            n197 = Greater Or Equal?(x=w386, y=u32 1750) -> (x >= y?=w385:bool)
            n198 = Select(t=SwerveRotationCalibrate."ResetQuad" ("Mode"), s=w385, f=SwerveRotationCalibrate."ManualHome" ("Mode")) -> (s? t:f=w389:T4)
            n199 = Bundle By Name(cluster=w380, "Mode"=w389, "Rotation Neutral Mode"=CTRE_Phoenix_MotorControl_NeutralMode."Override to Brake", "Rotation Control Mode"=w392, "Feedback Device"=w393) -> (w390:T8)
            n200 = call "SwerveHomeStore.vi"("Update?"=TRUE, "RearRightHomeIn"=w376, "RearLeftHomeIn"=w376, "FrontRightHomeIn"=w376, "FrontLeftHomeIn"=w376) -> ()  [unwired: 3 in, 4 out]
          }
          frame "ResetQuad" {
            w407 = T6 0 items=["PercentOutput"=0, "Position"=1, "Velocity"=2, "Current"=3, "Follower"=5, "MotionProfile"=6, "MotionMagic"=7, "MotionProfileArc"=10, "Disabled"=15] ("Rotation Control Mode")
            w406 = 0.0 ("P")
            # "Resets Quadrature encoders to 0 at the current encoder position"
            n201 = call "QuadEncActions.vi"("Zero?"=TRUE ("Reset?")) -> ()  [unwired: 7 in, 4 out]
            n202 = Bundle By Name(cluster=w410, "Mode"=SwerveRotationCalibrate."Drive", "Rotation Control Mode"=w407) -> (w409:T8)
            n203 = call "SwerveHomeStore.vi"() -> ("RearRightHomeOut"=w404:dbl, "RearLeftHomeOut"=w403:dbl, "FrontRightHomeOut"=w402:dbl, "FrontLeftHomeOut"=w401:dbl)  [unwired: 8 in]
          }
          frame "Drive" {
            w431 = T6 1 items=["PercentOutput"=0, "Position"=1, "Velocity"=2, "Current"=3, "Follower"=5, "MotionProfile"=6, "MotionMagic"=7, "MotionProfileArc"=10, "Disabled"=15] ("Rotation Control Mode")
            w433 = T7 0 items=["None"=-1, "QuadEncoder"=0, "Analog"=2, "Tachometer"=4, "Pulse Width Encoded Position"=8, "Sensor Sum (S0 + S1)"=9, "Sensor Difference (D0 - D1)"=10, "Remote Source 0"=11, "Remote Source 1"=12, "Software Emulated"=15] ("Feedback Device")
            # "Creates a deadband for all axes and inverts y-axis so that pushing the stick forward gives a positive value"
            n204 = Select(t=SwerveRotationCalibrate."Home" ("Mode"), s=w429, f=SwerveRotationCalibrate."Drive" ("Mode")) -> (s? t:f=w415:T4)
            n205 = Select(t=SwerveRotationCalibrate."ManualHome" ("Mode"), s=w413, f=w415) -> (s? t:f=w414:T4)
            n206 = call "SwerveMath.vi"("X-Axis"=w423, "Y-Axis"=w425, "Turn"=w424, "CentricToggle"=w411) -> ("FrontLeftAngle"=w435:dbl, "FrontLeftDrive"=w422:dbl, "FrontRightAngle"=w421:dbl, "FrontRightDrive"=w420:dbl, "RearLeftAngle"=w419:dbl, "RearLeftDrive"=w418:dbl, "RearRightAngle"=w417:dbl, "RearRightDrive"=w416:dbl)  [unwired: 16 in]
            n207 = call "QuadEncActions.vi"() -> ("RearRightQuadPos"=w439:i32, "RearLeftQuadPos"=w438:i32, "FrontRightQuadPos"=w440:i32, "FrontLeftQuadPos"=w436:i32)  [unwired: 8 in]
            n208 = Tick Count (ms)() -> (millisecond timer value=w426:u32)
            n209 = Bundle By Name(cluster=w434, "T0"=w426, "Mode"=w414, "Rotation Neutral Mode"=CTRE_Phoenix_MotorControl_NeutralMode."Override to Brake", "Rotation Control Mode"=w431, "Feedback Device"=w433) -> (w432:T8)
            n210 = call "SwerveWheelHeadingCalc.vi"("DriveIn"=w422, "Target"=w435, "Current"=w436) -> ("DriveOut"=w441:dbl, "TargetFinal"=w437:dbl)  [unwired: 7 in]
            n211 = call "SwerveWheelHeadingCalc.vi"("DriveIn"=w420, "Target"=w421, "Current"=w440) -> ("DriveOut"=w443:dbl, "TargetFinal"=w442:dbl)  [unwired: 7 in]
            n212 = call "SwerveWheelHeadingCalc.vi"("DriveIn"=w418, "Target"=w419, "Current"=w438) -> ("DriveOut"=w445:dbl, "TargetFinal"=w444:dbl)  [unwired: 7 in]
            n213 = call "SwerveWheelHeadingCalc.vi"("DriveIn"=w416, "Target"=w417, "Current"=w439) -> ("DriveOut"=w447:dbl, "TargetFinal"=w446:dbl)  [unwired: 7 in]
          }
        }
        n214 = call "SwerveDeadBand.vi"("FrontRightRotationIn"=w328, "FrontRightDriveIn"=w327, "RearLeftRotationIn"=w325, "RearLeftDriveIn"=w326, "FrontLeftDriveIn"=w329, "RearRightRotationIn"=w324, "FrontLeftRotationIn"=w330, "RearRightDriveIn"=w323, "RotationSettings"=w314) -> ("FrontLeftRotationOut"=w322:dbl, "FrontLeftDriveOut"=w321:dbl, "FrontRightRotationOut"=w320:dbl, "FrontRightDriveOut"=w319:dbl, "RearLeftRotationOut"=w318:dbl, "RearLeftDriveOut"=w317:dbl, "RearRightRotationOut"=w316:dbl, "RearRightDriveOut"=w315:dbl)  [unwired: 11 in]
        n215 = call "Drive_8CANSwerve.vi"("FrontLeftRotation"=w322, "FrontLeftDrive"=w321, "FrontRightRotation"=w320, "FrontRightDrive"=w319, "RearLeftRotation"=w318, "RearLeftDrive"=w317, "RearRightRotation"=w316, "RearRightDrive"=w315, "PIDInputs"=w334, "RotationSettings"=w314) -> ()  [unwired: 18 in]
      }
    }
    n216 = Wait (ms)(milliseconds to wait=w291) -> ()  [unwired: 1 out]
  }
  n217 = call <vilib>:"WPI_CompressorRefNum Registry Get.vi"("refnum name"="Compressor") -> ("CompressorDevRef"=w4:T18)  [unwired: 9 in, 1 out]
  n218 = while {
    tunnel: w4 -> [w450]
    stop <- w451 stop-if-true
    # "Pneumatics Compressor"
    n219 = call <vilib>:"WPI_CompressorStart.vi"("CompressorDevRef"=w450) -> ("CompressorDevRef"=w449:T18)  [unwired: 9 in, 1 out]
    n220 = call <vilib>:"WPI_CompressorGetEnableState.vi"("CompressorDevRef"=w449) -> ("error out"=w448:errorcluster)  [unwired: 1 in, 9 out]
    n221 = Unbundle By Name(w448) -> ("status"=w451:bool)
    n222 = Wait (ms)(milliseconds to wait=u32 100) -> ()  [unwired: 1 out]
  }
